vi "SRS 400 Read with options.vi"(3 "Instrument Address":refnum<visa-resource-name>, 4 "dwell source (int:0)":i32(slide) scale=0.0..1.0, 5 "dwell time":ext=0.002 format="%.4f", 6 "# periods":i32=10, 7 "count mode\n(a,b for t:0)":i16(slide) scale=0.0..2.0 scale format="%.2f") -> (0 "'B' data":dbl[](array[numeric]), 1 "'A' data":dbl[](array[numeric]), 2 "error":bool)   [LabVIEW 2020]
doc: "SR400 Read: If the count mode is set to \"A, B for T\", both counters will be active and two data arrays will be returned. Selecting \"A for T\" or \"A for B\" returns an array to the \" 'A' Data\" output only. The \"# Periods\" input sets the number of measurements made per scan (1 to 2000) and the \"Dwell Time\" sets the delay time between measurements (2E-3 to 60 seconds). If the \"Dwell Source\" is set to 'External', measurements are started with an externally supplied pulse at the \"Start\" input."
panel:
  in  "empty array":dbl[](array[numeric])
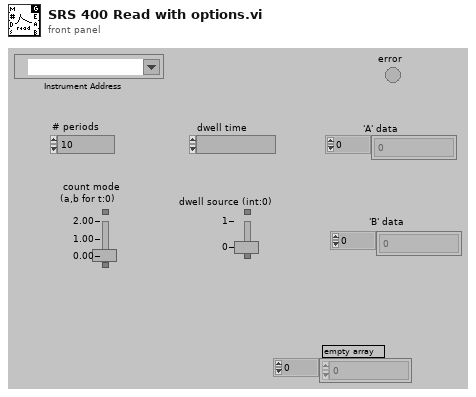
[diagram p1: front panel]
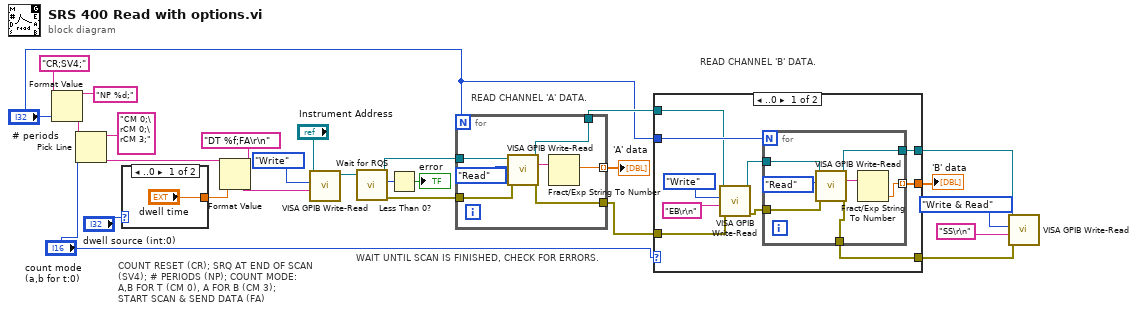
[diagram p0: block diagram]
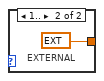
[diagram p2: hidden frame]
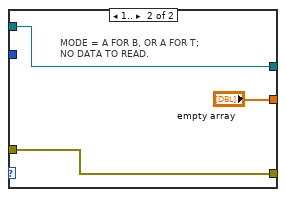
[diagram p3: hidden frame]
diagram:
  # "WAIT UNTIL SCAN IS FINISHED, CHECK FOR ERRORS."
  # "READ CHANNEL 'A' DATA."
  # "COUNT RESET (CR); SRQ AT END OF SCAN\n(SV4); # PERIODS (NP); COUNT MODE:\nA,B FOR T (CM 0), A FOR B (CM 3);\nSTART SCAN & SEND DATA (FA)"
  # "READ CHANNEL 'B' DATA."
  n1 = Format Value(string ("")="CR;SV4;", format string="NP %d;", value (0)="# periods") -> (output string=w12:string)
  n2 = Pick Line(string ("")=w12, multi-line string="CM 0;\rCM 0;\rCM 3;", line index="count mode\n(a,b for t:0)") -> (output string=w11:string)
  n3 = case shown="..0" "dwell source (int:0)" {
    tunnel: ["dwell time" ext 0.0] -> w14
    frame ..0 {
    }
    frame 1.. {
      # "EXTERNAL"
    }
  }
  n4 = Format Value(string ("")=w11, format string="DT %f;FA\r\n", value (0)=w14) -> (output string=w18:string)
  n5 = call "VISA GPIB Write-Read.vi"("Command"=w18, "Action"=enum16{"Write", "Read", "Write & Read"}."Write", "VISA resource name"="Instrument Address") -> ("dup VISA Session"=w3:refnum<visa-resource-name>)  [unwired: 5 in, 3 out]
  n6 = call <vilib>:"Wait for RQS.VI"("VISA resource name"=w3) -> ("error out"=w6:errorcluster, "status byte"=w7:u16, "VISA resource name out"=w5:refnum<visa-resource-name>)  [unwired: 8 in]
  n7 = Less Than 0?(x=w7) -> (x < 0?=→"error":bool)
  n8 = for {
    N: "# periods" -> [_]
    tunnel: [w35] -> w9 mode=indexing
    tunnel: [w32] -> w21
    tunnel: w6 -> [w31]
    tunnel: w5 -> [w30]
    tunnel: [w29] -> w4
    n9 = call "VISA GPIB Write-Read.vi"("error in (no error)"=w31, "Action"=enum16{"Write", "Read", "Write & Read"}."Read", "VISA resource name"=w30) -> ("error out"=w32:errorcluster, "String Returned"=w34:string, "dup VISA Session"=w29:refnum<visa-resource-name>)  [unwired: 5 in, 1 out]
    n10 = Fract/Exp String To Number(string=w34) -> (number=w35:dbl)  [unwired: 3 in, 1 out]
  }
  "'A' data" <- w9
  n11 = case shown="..0" "count mode\n(a,b for t:0)" {
    tunnel: [w42 "empty array"] -> w22
    tunnel: "# periods" -> [w41 _]
    tunnel: w4 -> [w39 w54]
    tunnel: [w40 w53] -> w25
    tunnel: [w37 w54] -> w26
    tunnel: w21 -> [w36 w53]
    frame ..0 {
      n12 = call "VISA GPIB Write-Read.vi"("error in (no error)"=w36, "Command"="EB\r\n", "Action"=enum16{"Write", "Read", "Write & Read"}."Write", "VISA resource name"=w39) -> ("error out"=w45:errorcluster, "dup VISA Session"=w38:refnum<visa-resource-name>)  [unwired: 4 in, 2 out]
      n13 = for {
        N: w41 -> [_]
        tunnel: [w52] -> w42 mode=indexing
        tunnel: w45 -> [w49]
        tunnel: w38 -> [w47]
        tunnel: [w48] -> w40
        tunnel: [w46] -> w37
        n14 = call "VISA GPIB Write-Read.vi"("error in (no error)"=w49, "Action"=enum16{"Write", "Read", "Write & Read"}."Read", "VISA resource name"=w47) -> ("error out"=w48:errorcluster, "String Returned"=w51:string, "dup VISA Session"=w46:refnum<visa-resource-name>)  [unwired: 5 in, 1 out]
        n15 = Fract/Exp String To Number(string=w51) -> (number=w52:dbl)  [unwired: 3 in, 1 out]
      }
    }
    frame 1.. {
      # "MODE = A FOR B, OR A FOR T; \nNO DATA TO READ."
    }
  }
  "'B' data" <- w22
  n16 = call "VISA GPIB Write-Read.vi"("error in (no error)"=w25, "Command"="SS\r\n", "Action"=enum16{"Write", "Read", "Write & Read"}."Write & Read", "VISA resource name"=w26) -> ()  [unwired: 4 in, 4 out]
